vi "Send Software Trigger [SWT] Core.vi"(8 "error in (no error)":errorcluster, 11 "CS++DCPwr in":refnum<class "CS++DCPwr.lvclass">) -> (0 "error out":errorcluster, 3 "CS++DCPwr out":refnum<class "CS++DCPwr.lvclass">)   [LabVIEW 2013, in "CS++DCPwr.lvlib" / "CS++DCPwr.lvclass"]
doc: "This VI sends a command to trigger the power supply. Call this VI if you configure the power supply to respond to software triggers. If the power supply is not configured to respond to software triggers, this VI returns the error IVIDCPWR_ERROR_TRIGGER_NOT_SOFTWARE (0xBFFA1001).\n\nNotes:\n\n(1) This VI is part of the IviDCPwrSoftwareTrigger [SWT] extension group."
uses:
  CS++DCPwr.lvclass
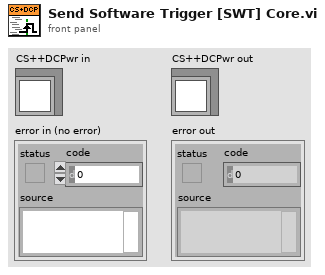
[diagram p1: front panel]
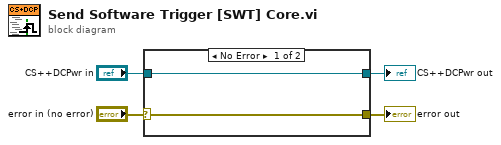
[diagram p0: block diagram]
diagram:
  n1 = case shown="No Error" "error in (no error)" {
    selector: "error in (no error)" -> [w5 w8]
    tunnel: [w5 w8] -> w3
    tunnel: [w6 w7] -> w1
    tunnel: "CS++DCPwr in" -> [w6 w7]
    frame No Error {
    }
    frame Error {
    }
  }
  "error out" <- w3
  "CS++DCPwr out" <- w1
